vi "CRYCalc Wave & Wave.vi"(8 "Wave in_2":T1={"Waveform"={"X0"=0.0, "dX"=0.0, "Y"=[]}, "X data"=1, "Y data"=1, "Y axis"=1, "X unit"="s", "Y unit"="V", "Y dB ref"=1.0, "display Y"=TRUE, "display X"=TRUE, "Overload?"=FALSE, "Test Info"="", "Step No."=0, "Name"="", "protected"=FALSE, "Sqc history"=[], "Signal Channel ID"=0, "Plot Settings"={"Color"=0, "Interpolation"=0, "Point Style"=0, "Line Style"=0, "Point Color"=0, "Line Width"=0, "Bar Plot Style"=0, "Fill To"=0}, "AutoProtect"=FALSE} {"Y dB ref" format="%.1f"; "Y axis" items=["Log", "Lin"]; "Y data" items=["dB", "Lin"]; "X data" items=["dB", "Lin"]}, 9 "Work in":u16(slide), 10 "Operator":u16(ring) items=["+", "--", "x", "/"], 11 "Wave in_1":T1={"Waveform"={"X0"=0.0, "dX"=0.0, "Y"=[]}, "X data"=1, "Y data"=1, "Y axis"=1, "X unit"="s", "Y unit"="V", "Y dB ref"=1.0, "display Y"=TRUE, "display X"=TRUE, "Overload?"=FALSE, "Test Info"="", "Step No."=0, "Name"="", "protected"=FALSE, "Sqc history"=[], "Signal Channel ID"=0, "Plot Settings"={"Color"=0, "Interpolation"=0, "Point Style"=0, "Line Style"=0, "Point Color"=0, "Line Width"=0, "Bar Plot Style"=0, "Fill To"=0}, "AutoProtect"=FALSE} {"Y dB ref" format="%.1f"; "Y axis" items=["Log", "Lin"]; "Y data" items=["dB", "Lin"]; "X data" items=["dB", "Lin"]}) -> (3 "Wave out":T1={"Waveform"={"X0"=0.0, "dX"=0.0, "Y"=[]}, "X data"=1, "Y data"=1, "Y axis"=1, "X unit"="s", "Y unit"="V", "Y dB ref"=1.0, "display Y"=TRUE, "display X"=TRUE, "Overload?"=FALSE, "Test Info"="", "Step No."=0, "Name"="", "protected"=FALSE, "Sqc history"=[], "Signal Channel ID"=0, "Plot Settings"={"Color"=0, "Interpolation"=0, "Point Style"=0, "Line Style"=0, "Point Color"=0, "Line Width"=0, "Bar Plot Style"=0, "Fill To"=0}, "AutoProtect"=FALSE} {"Y dB ref" format="%.1f"; "Y axis" items=["Log", "Lin"]; "Y data" items=["dB", "Lin"]; "X data" items=["dB", "Lin"]})   [LabVIEW 2013]
uses:
  Typedef Control/CRYWaveform Cluster.ctl
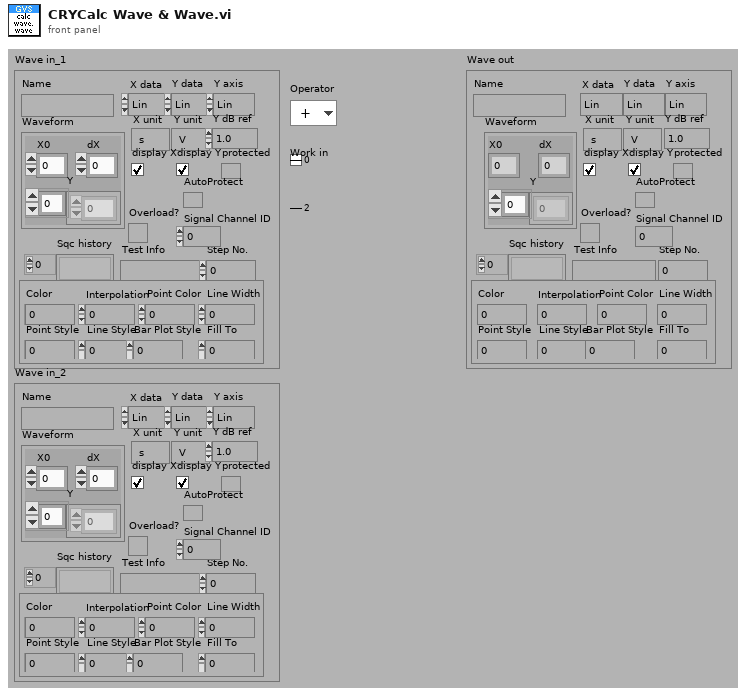
[diagram p1: front panel]
types:
  T1 = typedef "CRYWaveform Cluster.ctl" = cluster{"Waveform":cluster{"X0":dbl, "dX":dbl, "Y":sgl[]}, "X data":u16, "Y data":u16, "Y axis":u16, "X unit":string, "Y unit":string, "Y dB ref":dbl, "display Y":bool, "display X":bool, "Overload?":bool, "Test Info":string, "Step No.":i32, "Name":string, "protected":bool, "Sqc history":string[], "Signal Channel ID":i32, "Plot Settings":cluster{"Color":u32, "Interpolation":u8, "Point Style":u8, "Line Style":u8, "Point Color":u32, "Line Width":u8, "Bar Plot Style":u8, "Fill To":i16}, "AutoProtect":bool}
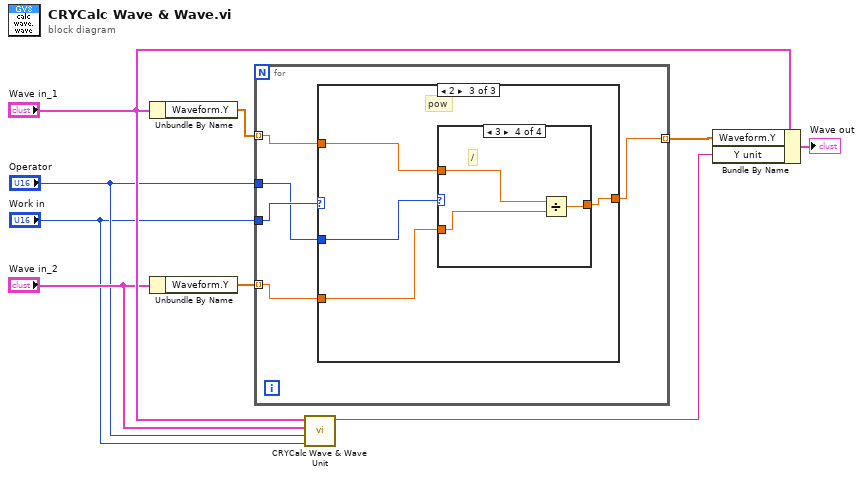
[diagram p0: block diagram]
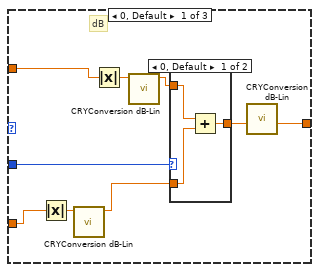
[diagram p2: hidden frame]
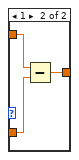
[diagram p3: hidden frame]
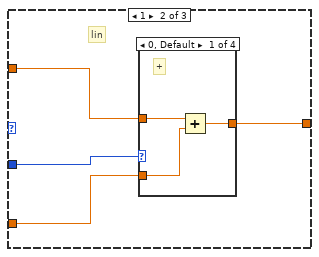
[diagram p4: hidden frame]
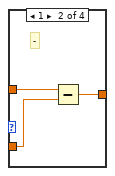
[diagram p5: hidden frame]
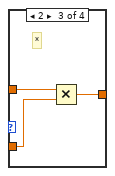
[diagram p6: hidden frame]
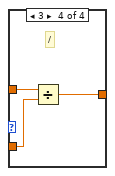
[diagram p7: hidden frame]
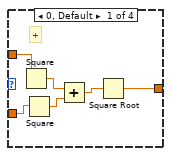
[diagram p8: hidden frame]
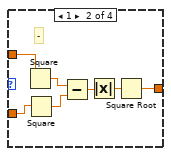
[diagram p9: hidden frame]
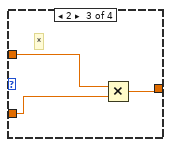
[diagram p10: hidden frame]
diagram:
  n1 = Unbundle By Name("Wave in_1") -> ("Waveform.Y"=w9:sgl[])
  n2 = Unbundle By Name("Wave in_2") -> ("Waveform.Y"=w7:sgl[])
  n3 = for {
    tunnel: "Operator" -> [w13]
    tunnel: w9 -> [w11] mode=indexing
    tunnel: "Work in" -> [w14]
    tunnel: w7 -> [w12] mode=indexing
    tunnel: [w10] -> w1 mode=indexing
    n4 = case shown="2" w14 {
      tunnel: w13 -> [w23 w33 w49]
      tunnel: w12 -> [w17 w31 w48]
      tunnel: w11 -> [w19 w32 w47]
      tunnel: [w18 w30 w46] -> w10
      frame 0, Default {
        # "dB"
        n5 = Absolute Value(x=w17) -> (abs(x)=w15:sgl)
        n6 = call "CRYConversion dB-Lin.vi"("Lin In"=w15) -> ("Log Out"=w16:dbl)  [unwired: 5 in, 3 out]
        n7 = Absolute Value(x=w19) -> (abs(x)=w20:sgl)
        n8 = call "CRYConversion dB-Lin.vi"("Lin In"=w20) -> ("Log Out"=w21:dbl)  [unwired: 5 in, 3 out]
        n9 = case shown="0, Default" w23 {
          tunnel: w16 -> [w25 w27]
          tunnel: w21 -> [w26 w28]
          tunnel: [w24 w29] -> w22
          frame 0, Default {
            n10 = Add(x=w26, y=w25) -> (x+y=w24:dbl)
          }
          frame 1 {
            n11 = Subtract(x=w28, y=w27) -> (x-y=w29:dbl)
          }
        }
        n12 = call "CRYConversion dB-Lin.vi"("Log In"=w22) -> ("Lin Out"=w18:dbl)  [unwired: 5 in, 3 out]
      }
      frame 1 {
        # "lin"
        n13 = case shown="0, Default" w33 {
          tunnel: w32 -> [w36 w39 w42 w44]
          tunnel: w31 -> [w35 w38 w41 w43]
          tunnel: [w34 w37 w40 w45] -> w30
          frame 0, Default {
            # "+"
            n14 = Add(x=w36, y=w35) -> (x+y=w34:sgl)
          }
          frame 1 {
            # "-"
            n15 = Subtract(x=w39, y=w38) -> (x-y=w37:sgl)
          }
          frame 2 {
            # "*"
            n16 = Multiply(x=w42, y=w41) -> (x*y=w40:sgl)
          }
          frame 3 {
            # "/"
            n17 = Divide(x=w44, y=w43) -> (x/y=w45:sgl)
          }
        }
      }
      frame 2 {
        # "pow"
        n18 = case shown="3" w49 {
          tunnel: w47 -> [w55 w62 w64 w67]
          tunnel: w48 -> [w54 w61 w63 w66]
          tunnel: [w50 w56 w65 w68] -> w46
          frame 0, Default {
            # "+"
            n19 = Square(x=w55) -> (x^2=w53:sgl)
            n20 = Square(x=w54) -> (x^2=w52:sgl)
            n21 = Add(x=w53, y=w52) -> (x+y=w51:sgl)
            n22 = Square Root(x=w51) -> (sqrt(x)=w50:sgl)
          }
          frame 1 {
            # "-"
            n23 = Square(x=w62) -> (x^2=w60:sgl)
            n24 = Square(x=w61) -> (x^2=w59:sgl)
            n25 = Subtract(x=w60, y=w59) -> (x-y=w58:sgl)
            n26 = Absolute Value(x=w58) -> (abs(x)=w57:sgl)
            n27 = Square Root(x=w57) -> (sqrt(x)=w56:sgl)
          }
          frame 2 {
            # "*"
            n28 = Multiply(x=w64, y=w63) -> (x*y=w65:sgl)
          }
          frame 3 {
            # "/"
            n29 = Divide(x=w67, y=w66) -> (x/y=w68:sgl)
          }
        }
      }
    }
  }
  n30 = call "CRYCalc Wave & Wave Unit.vi"("Work in"="Work in", "Operator"="Operator", "Wave in_2"="Wave in_2", "Wave in_1"="Wave in_1") -> ("Y unit"=w2:string)  [unwired: 4 in, 3 out]
  n31 = Bundle By Name(cluster="Wave in_1", "Waveform.Y"=w1, "Y unit"=w2) -> (→"Wave out":T1)
